vi "2 MissionHeadingGoodness.vi"(2 "Heading":dbl) -> (6 "Target Goodness":dbl, 7 "No-Go Goodness":dbl, 9 "Direction Change Goodness":dbl)   [LabVIEW 2011]
doc: "This VI simply runs the necessary components of the goodness function and outputs their \"goodness value\" for a specific test heading."
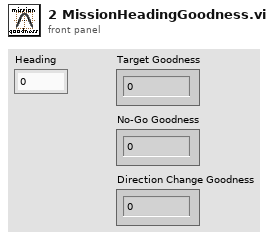
[diagram p1: front panel]
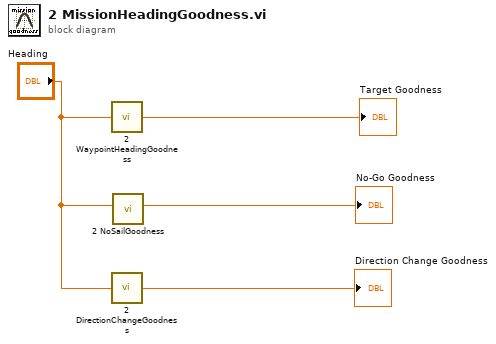
[diagram p0: block diagram]
diagram:
  n1 = call "2 WaypointHeadingGoodness.vi"("Heading to Test"="Heading") -> ("Goodness"=→"Target Goodness":dbl)  [unwired: 4 in]
  n2 = call "2 DirectionChangeGoodness.vi"("Test Heading"="Heading") -> ("Goodness"=→"Direction Change Goodness":dbl)
  n3 = call "2 NoSailGoodness.vi"("Heading to Test"="Heading") -> ("Goodness"=→"No-Go Goodness":dbl)  [unwired: 10 in]
